vi "DSF.Shared.Constants.vi"   [LabVIEW 2017, in "DSF.Engine.lvlib"]
uses:
  DSF.Engine.lvlib
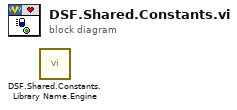
[diagram p0: block diagram]
diagram:
  n1 = call "DSF.Shared.Constants.Library Name.Engine.vi"() -> ()  [unwired: 11 in, 1 out]
